vi "1A_AnalyzePulseTrain.vi"(0 "Waveform In":waveform(dbl)={"t0"=timestamp(3433165898.5470004 s since 1904-01-01), "dt"=1e-05, "Y"=array[4250 elements]}, 5 "Repetitions in the Input Waveform":i32, 7 "Pulse Characteristics":T2={"Pulses per Cycle"=2, "Load Resistance (Ohms)"=750.0, "Krec Value"=2, "Recovery Mode (T=Active)"=TRUE, "Target Stim Currents (Amps)"=[]}) -> (2 "Avg. CBC Width":dbl format="%0.6f", 3 "Avg. CBC Amplitude":dbl format="%0.2f", 4 "Stim PW":dbl[](array[numeric]), 6 "Stim Amplitude":dbl[](array[numeric]), 8 "Interphase Delay":dbl[](array[numeric]) format="%#.6g", 10 "Recovery PW":dbl[](array[numeric]), 12 "Waveform Parameters":T1, 13 "Frequency":dbl, 14 "Recovery Holdoff":dbl[](array[numeric]), 15 "Recovery Amplitude":dbl[](array[numeric]))   [LabVIEW 2010]
uses:
  Pulse Train Parameters.ctl
  <vilib>/measure/mamon.llb/Trigger Detection for 1 Channel.vi
  <vilib>/measure/NI_MAPro.lvlib
  <vilib>/Analysis/NI_AALBase.lvlib
panel:
  out "Normalized Waveform":waveform(dbl)(graph)
  # "The input waveform should be a capture of the STIM chip output\n(before the cap) when the output is held at 1/2 HVDD by the\nLoad Resistance.  This ensures that passive recovery and CBC\npulses are captured, because they look like pulses pulled to GND."
  # "The elements in these arrays correspond to the pulses per cycle.\nThey are the averages over all the repetitions in the waveform."
  # "Enter Target Current\nfor each in array below"
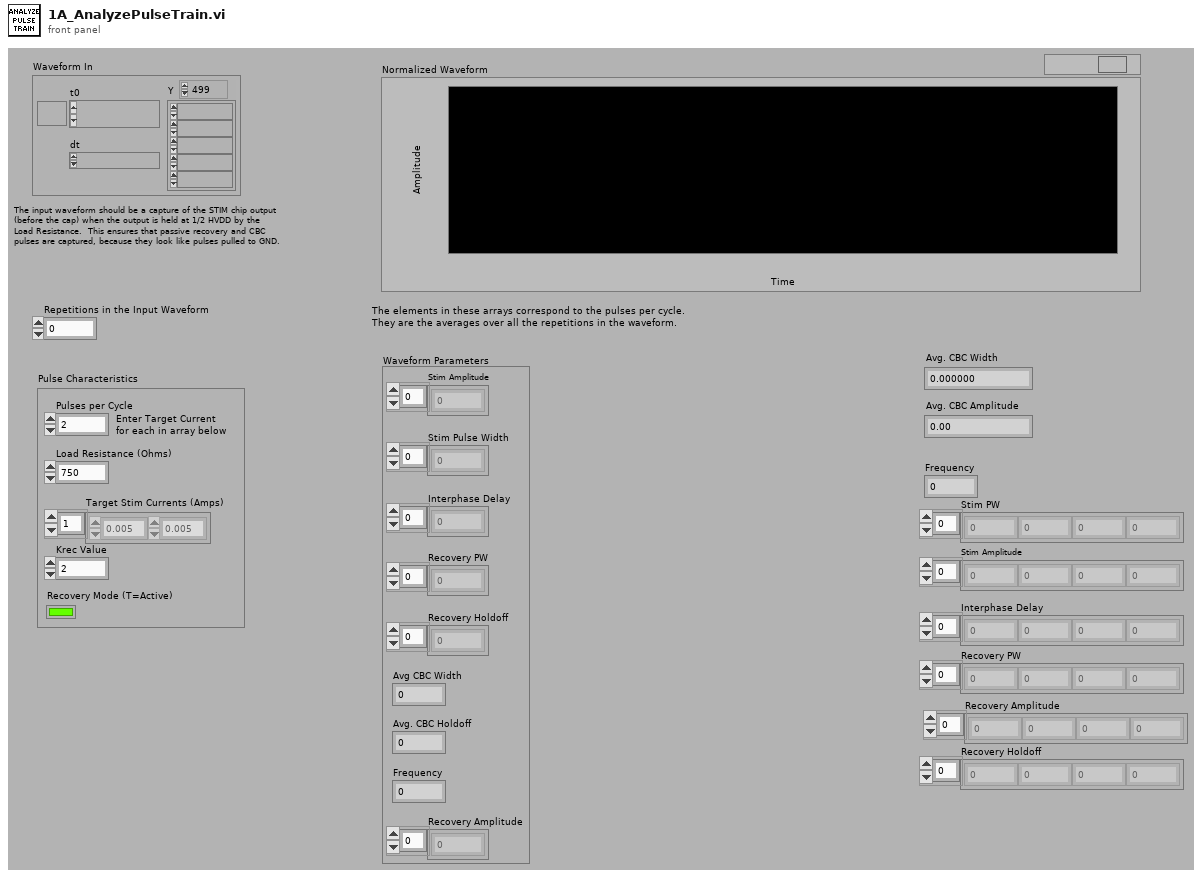
[diagram p1: front panel]
types:
  T1 = typedef "Pulse Train Parameters.ctl" = cluster{"Stim Amplitude":dbl[], "Stim Pulse Width":dbl[], "Interphase Delay":dbl[], "Recovery PW":dbl[], "Recovery Holdoff":dbl[], "Avg CBC Width":dbl, "Frequency":dbl, "Avg. CBC Holdoff":dbl, "Recovery Amplitude":dbl[]}
  T2 = cluster{"Pulses per Cycle":i32, "Load Resistance (Ohms)":dbl, "Krec Value":i32, "Recovery Mode (T=Active)":bool, "Target Stim Currents (Amps)":dbl[]}
  T3 = cluster{"trigger slope":u16, "Trigger Level":dbl}[]
  T4 = cluster{"trigger slope":u16, "Trigger Level":dbl}
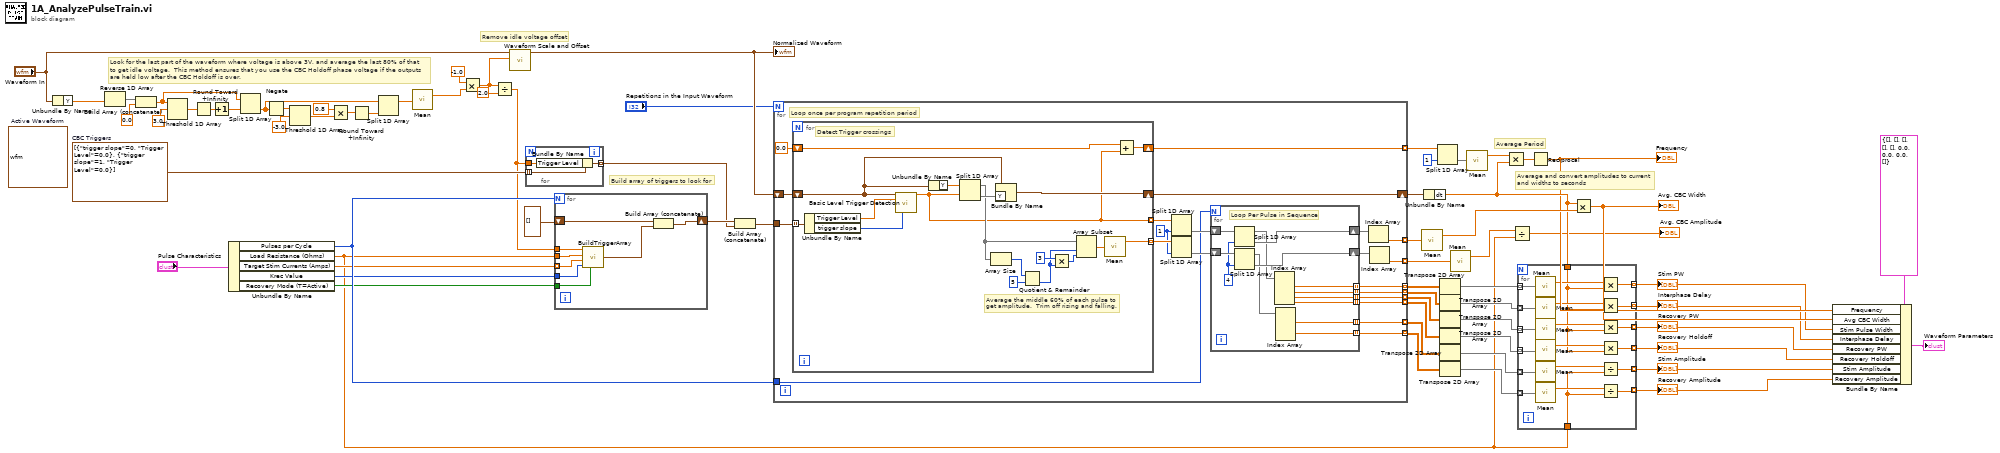
[diagram p0: block diagram]
diagram:
  (unwired) waveform(dbl) {"t0"=timestamp(3418839276.250478 s since 1904-01-01), "dt"=1e-06, "Y"=[5.0, 5.0, 9.0, 9.0, 9.0, 9.0, 9.0, 9.0, 9.0, 9.0, 5.0, 5.0, 5.0, 3.0, 3.0, 3.0, 3.0, 3.0, 3.0, 3.0, 3.0, 3.0, 3.0, 3.0, 3.0, 3.0, 3.0, 3.0, 3.0, 5.0, 5.0, 5.0, 5.0, 8.0, 8.0, 8.0, 8.0, 8.0, 8.0, 8.0, 8.0, 5.0, 5.0, 5.0, 3.0, 3.0, 3.0, 3.0, 3.0, 3.0, 3.0, 3.0, 3.0, 3.0, 3.0, 3.0, 3.0, 3.0, 3.0, 3.0, 5.0, 5.0, 5.0, 5.0, 0.0, 0.0, 0.0, 0.0, 0.0, 5.0, 5.0, 5.0, 5.0, 5.0, 5.0, 5.0, 5.0, 5.0, 5.0, 5.0, 5.0, 5.0, 5.0, 5.0, 5.0, 5.0, 5.0, 5.0, 5.0, 5.0, 5.0, 5.0, 5.0, 5.0, 5.0, 5.0, 5.0, 5.0, 5.0, 5.0, 5.0, 5.0, 9.0, 9.0, 9.0, 9.0, 9.0, 9.0, 9.0, 9.0, 5.0, 5.0, 5.0, 3.0, 3.0, 3.0, 3.0, 3.0, 3.0, 3.0, 3.0, 3.0, 3.0, 3.0, 3.0, 3.0, 3.0, 3.0, 3.0, 5.0, 5.0, 5.0, 5.0, 8.0, 8.0, 8.0, 8.0, 8.0, 8.0, 8.0, 8.0, 5.0, 5.0, 5.0, 3.0, 3.0, 3.0, 3.0, 3.0, 3.0, 3.0, 3.0, 3.0, 3.0, 3.0, 3.0, 3.0, 3.0, 3.0, 3.0, 5.0, 5.0, 5.0, 5.0, 0.0, 0.0, 0.0, 0.0, 0.0, 5.0, 5.0, 5.0, 5.0, 5.0, 5.0, 5.0, 5.0, 5.0, 5.0, 5.0, 5.0, 5.0, 5.0, 5.0, 5.0, 5.0, 5.0, 5.0, 5.0, 5.0, 5.0, 5.0, 5.0, 5.0, 5.0, 5.0, 5.0, 5.0, 5.0, 5.0, 5.0, 5.0, 9.0, 9.0, 9.0, 9.0, 9.0, 9.0, 9.0, 9.0, 5.0, 5.0, 5.0, 3.0, 3.0, 3.0, 3.0, 3.0, 3.0, 3.0, 3.0, 3.0, 3.0, 3.0, 3.0, 3.0, 3.0, 3.0, 3.0, 5.0, 5.0, 5.0, 5.0, 8.0, 8.0, 8.0, 8.0, 8.0, 8.0, 8.0, 8.0, 5.0, 5.0, 5.0, 3.0, 3.0, 3.0, 3.0, 3.0, 3.0, 3.0, 3.0, 3.0, 3.0, 3.0, 3.0, 3.0, 3.0, 3.0, 3.0, 5.0, 5.0, 5.0, 5.0, 0.0, 0.0, 0.0, 0.0, 0.0, 5.0, 5.0, 5.0, 5.0, 5.0, 5.0, 5.0, 5.0, 5.0, 5.0, 5.0, 5.0, 5.0, 5.0, 5.0, 5.0, 5.0, 5.0, 5.0, 5.0, 5.0, 5.0, 5.0, 5.0, 5.0, 5.0, 5.0, 5.0, 5.0, 5.0, 5.0, 5.0, 5.0, 9.0, 9.0, 9.0, 9.0, 9.0, 9.0, 9.0, 9.0, 5.0, 5.0, 5.0, 3.0, 3.0, 3.0, 3.0, 3.0, 3.0, 3.0, 3.0, 3.0, 3.0, 3.0, 3.0, 3.0, 3.0, 3.0, 3.0, 5.0, 5.0, 5.0, 5.0, 8.0, 8.0, 8.0, 8.0, 8.0, 8.0, 8.0, 8.0, 5.0, 5.0, 5.0, 3.0, 3.0, 3.0, 3.0, 3.0, 3.0, 3.0, 3.0, 3.0, 3.0, 3.0, 3.0, 3.0, 3.0, 3.0, 3.0, 5.0, 5.0, 5.0, 5.0, 0.0, 0.0, 0.0, 0.0, 0.0, 5.0, 5.0, 5.0, 5.0, 5.0, 5.0, 5.0, 5.0, 5.0, 5.0, 5.0, 5.0, 5.0, 5.0, 5.0, 5.0, 5.0, 5.0, 5.0, 5.0, 5.0, 5.0, 5.0, 5.0, 5.0, 5.0, 5.0, 5.0, 5.0, 5.0, 5.0, 5.0, 5.0, 9.0, 9.0, 9.0, 9.0, 9.0, 9.0, 9.0, 9.0, 5.0, 5.0, 5.0, 3.0, 3.0, 3.0, 3.0, 3.0, 3.0, 3.0, 3.0, 3.0, 3.0, 3.0, 3.0, 3.0, 3.0, 3.0, 3.0, 5.0, 5.0, 5.0, 5.0, 8.0, 8.0, 8.0, 8.0, 8.0, 8.0, 8.0, 8.0, 5.0, 5.0, 5.0, 3.0, 3.0, 3.0, 3.0, 3.0, 3.0, 3.0, 3.0, 3.0, 3.0, 3.0, 3.0, 3.0, 3.0, 3.0, 3.0, 5.0, 5.0, 5.0, 5.0, 0.0, 0.0, 0.0, 0.0, 0.0, 5.0, 5.0, 5.0, 5.0, 5.0, 5.0, 5.0, 5.0, 5.0, 5.0, 5.0, 5.0, 5.0, 5.0, 5.0, 5.0, 5.0, 5.0, 5.0, 5.0, 5.0, 5.0, 5.0, 5.0, 5.0, 5.0, 5.0, 5.0, 5.0, 5.0, 5.0, 5.0, 5.0, 5.0]}  # Active Waveform
  w64 = T3 [{"trigger slope"=0, "Trigger Level"=0.0}, {"trigger slope"=1, "Trigger Level"=0.0}]  # CBC Triggers
  # "Look for the last part of the waveform where voltage is above 3V, and average the last 80% of that\nto get idle voltage.  This method ensures that you use the CBC Holdoff phase voltage if the outputs\nare held low after the CBC Holdoff is over."
  # "Average Period"
  # "Average and convert amplitudes to current\nand widths to seconds"
  # "Build array of triggers to look for"
  # "Remove idle voltage offset"
  n1 = Unbundle By Name("Waveform In") -> ("Y"=w2:dbl[])
  n2 = Reverse 1D Array(array=w2) -> (reversed array=w17:dbl[])
  n3 = Build Array (concatenate)(w17, 0.0 ("y")) -> (w12:dbl[])
  n4 = Threshold 1D Array(2:3.0 ("y"), 3:w12) -> (0:w14:dbl)  [unwired: 1 in]
  n5 = Round Toward +Infinity(x=w14) -> (ceil(x): smallest int >= x=w13:dbl)
  n6 = Increment(x=w13) -> (x+1=w3:dbl)
  n7 = Unbundle By Name("Pulse Characteristics") -> ("Pulses per Cycle"=w44:i32, "Load Resistance (Ohms)"=w35:dbl, "Target Stim Currents (Amps)"=w41:dbl[], "Krec Value"=w40:i32, "Recovery Mode (T=Active)"=w42:bool)
  n8 = Split 1D Array(array=w12, index=w3) -> (second subarray=w5:dbl[])  [unwired: 1 out]
  n9 = Negate(x=w5) -> (-x=w10:dbl[])
  n10 = Threshold 1D Array(2:-3.0 ("y"), 3:w10) -> (0:w9:dbl)  [unwired: 1 in]
  n11 = Multiply(x=0.8, y=w9) -> (x*y=w7:dbl)
  n12 = Round Toward +Infinity(x=w7) -> (ceil(x): smallest int >= x=w6:dbl)
  n13 = Split 1D Array(array=w5, index=w6) -> (first subarray=w4:dbl[])  [unwired: 1 out]
  n14 = call <vilib>:"Mean.vi"("X"=w4) -> ("mean"=w1:dbl)  [unwired: 1 out]
  n15 = Multiply(x=-1.0, y=w1) -> (x*y=w63:dbl)
  n16 = Divide(x=w63, y=2.0) -> (x/y=w43:dbl)
  n17 = call <vilib>:"Waveform Scale and Offset.vi"("offset"=w63, "waveform in"="Waveform In") -> ("waveform out"=w59:waveform(dbl))  [unwired: 8 in, 1 out]
  "Normalized Waveform" <- w59
  n18 = for {
    tunnel: w64 -> [w72] mode=indexing
    tunnel: w43 -> [w71]
    tunnel: [w70] -> w61 mode=indexing
    n19 = Bundle By Name(cluster=w72, "Trigger Level"=w71) -> (w70:T4)
  }
  n20 = for {
    N: w44 -> [_]
    shift-right: [w80] -> w65
    shift-left: T3 [] -> [w79]
    tunnel: w43 -> [w78]
    tunnel: w42 -> [w77]
    tunnel: w35 -> [w76]
    tunnel: w41 -> [w75] mode=indexing
    tunnel: w40 -> [w74]
    n21 = call "BuildTriggerArray.vi"("CBC Trigger Level"=w78, "Load Resistance (Ohms)"=w76, "Target Stim Current (Amps)"=w75, "Krec Value"=w74, "Recovery Mode (T=Active)"=w77) -> ("Pulse Triggers"=w73:T3)
    n22 = Build Array (concatenate)(w79, w73) -> (w80:T3)
  }
  n23 = Build Array (concatenate)(w65, w61) -> (w60:T3)
  n24 = for {
    N: "Repetitions in the Input Waveform" -> [_]
    tunnel: w60 -> [w101]
    shift-right: [w97] -> w38
    shift-left: w59 -> [w100]
    tunnel: w44 -> [w94]
    tunnel: [w91] -> w58 mode=indexing
    tunnel: [w90] -> w57 mode=indexing
    tunnel: [w89] -> w56 mode=indexing
    tunnel: [w88] -> w55 mode=indexing
    tunnel: [w87] -> w54 mode=indexing
    tunnel: [w86] -> w53 mode=indexing
    tunnel: [w85] -> w52 mode=indexing
    tunnel: [w84] -> w51 mode=indexing
    tunnel: [w81] -> w34 mode=indexing
    w98 = 1 ("index")
    # "Loop once per program repetition period"
    n25 = for {
      tunnel: w101 -> [w132] mode=indexing
      shift-right: [w118] -> w97
      shift-left: w100 -> [w127]
      tunnel: [w119] -> w99 mode=indexing
      tunnel: [w115] -> w82 mode=indexing
      shift-right: [w117] -> w81
      shift-left: 0.0 -> [w116]
      # "Detect Trigger crossings"
      # "Average the middle 60% of each pulse to\nget amplitude.  Trim off rising and falling."
      n26 = Unbundle By Name(w132) -> ("Trigger Level"=w131:dbl, "trigger slope"=w130:u16)
      n27 = call-poly <vilib>:"Basic Level Trigger Detection.vi"("signal in"=w127, "level"=w131, "trigger slope"=w130) -> ("trigger location"=w115:dbl)  [unwired: 10 in, 2 out]
      n28 = Unbundle By Name(w127) -> ("Y"=w129:dbl[])
      n29 = Split 1D Array(array=w129, index=w115) -> (first subarray=w121:dbl[], second subarray=w128:dbl[])
      n30 = Array Size(array=w121) -> (size(s)=w126:i32)
      n31 = Bundle By Name(cluster=w127, "Y"=w128) -> (w118:waveform(dbl))
      n32 = Quotient & Remainder(x=w126, y=5) -> (floor(x/y)=w123:i32)  [unwired: 1 out]
      n33 = Multiply(x=3, y=w123) -> (x*y=w122:i32)
      n34 = Array Subset(array=w121, index=w123, length=w122) -> (w120:dbl[])
      n35 = call <vilib>:"Mean.vi"("X"=w120) -> ("mean"=w119:dbl)  [unwired: 1 out]
      n36 = Add(x=w116, y=w115) -> (x+y=w117:dbl)
    }
    n37 = Split 1D Array(array=w82, index=w98) -> (second subarray=w96:dbl[])  [unwired: 1 out]
    n38 = Split 1D Array(array=w99, index=w98) -> (second subarray=w95:dbl[])  [unwired: 1 out]
    n39 = for {
      N: w94 -> [_]
      shift-right: [w112] -> w93
      shift-left: w96 -> [w114]
      shift-right: [w111] -> w92
      shift-left: w95 -> [w113]
      tunnel: [w108] -> w89 mode=indexing
      tunnel: [w107] -> w88 mode=indexing
      tunnel: [w106] -> w87 mode=indexing
      tunnel: [w105] -> w86 mode=indexing
      tunnel: [w104] -> w85 mode=indexing
      tunnel: [w103] -> w84 mode=indexing
      w102 = 4 ("index")
      # "Loop Per Pulse in Sequence"
      n40 = Split 1D Array(array=w114, index=w102) -> (first subarray=w110:dbl[], second subarray=w112:dbl[])
      n41 = Split 1D Array(array=w113, index=w102) -> (first subarray=w109:dbl[], second subarray=w111:dbl[])
      n42 = Index Array(array=w110) -> (element #1=w108:dbl, element #2=w107:dbl, element #3=w106:dbl, element #4=w105:dbl)  [unwired: 4 in]
      n43 = Index Array(array=w109) -> (element #1=w104:dbl, element #3=w103:dbl)  [unwired: 4 in, 2 out]
    }
    n44 = Index Array(array=w93) -> (element=w91:dbl)  [unwired: 1 in]
    n45 = Index Array(array=w92) -> (element=w90:dbl)  [unwired: 1 in]
  }
  n46 = call <vilib>:"Mean.vi"("X"=w58) -> ("mean"=w37:dbl)  [unwired: 1 out]
  n47 = Unbundle By Name(w38) -> ("dt"=w31:dbl)
  n48 = Split 1D Array(array=w34, index=1) -> (second subarray=w33:dbl[])  [unwired: 1 out]
  n49 = Transpose 2D Array(2D array=w56) -> (transposed array=w50:dbl[][])
  n50 = Transpose 2D Array(2D array=w55) -> (transposed array=w49:dbl[][])
  n51 = Transpose 2D Array(2D array=w54) -> (transposed array=w48:dbl[][])
  n52 = Transpose 2D Array(2D array=w53) -> (transposed array=w47:dbl[][])
  n53 = Transpose 2D Array(2D array=w52) -> (transposed array=w46:dbl[][])
  n54 = Transpose 2D Array(2D array=w51) -> (transposed array=w45:dbl[][])
  n55 = call <vilib>:"Mean.vi"("X"=w57) -> ("mean"=w36:dbl)  [unwired: 1 out]
  n56 = call <vilib>:"Mean.vi"("X"=w33) -> ("mean"=w32:dbl)  [unwired: 1 out]
  n57 = Multiply(x=w32, y=w31) -> (x*y=w30:dbl)
  n58 = Divide(x=w36, y=w35) -> (x/y=→"Avg. CBC Amplitude":dbl)
  n59 = for {
    tunnel: w50 -> [w152] mode=indexing
    tunnel: w49 -> [w151] mode=indexing
    tunnel: w48 -> [w150] mode=indexing
    tunnel: w47 -> [w149] mode=indexing
    tunnel: w46 -> [w148] mode=indexing
    tunnel: w45 -> [w147] mode=indexing
    tunnel: [w146] -> w24 mode=indexing
    tunnel: [w145] -> w23 mode=indexing
    tunnel: [w144] -> w22 mode=indexing
    tunnel: [w143] -> w21 mode=indexing
    tunnel: [w142] -> w20 mode=indexing
    tunnel: [w141] -> w19 mode=indexing
    tunnel: w31 -> [w134]
    tunnel: w35 -> [w133]
    n60 = call <vilib>:"Mean.vi"("X"=w152) -> ("mean"=w139:dbl)  [unwired: 1 out]
    n61 = call <vilib>:"Mean.vi"("X"=w151) -> ("mean"=w138:dbl)  [unwired: 1 out]
    n62 = call <vilib>:"Mean.vi"("X"=w150) -> ("mean"=w137:dbl)  [unwired: 1 out]
    n63 = call <vilib>:"Mean.vi"("X"=w149) -> ("mean"=w136:dbl)  [unwired: 1 out]
    n64 = call <vilib>:"Mean.vi"("X"=w148) -> ("mean"=w135:dbl)  [unwired: 1 out]
    n65 = call <vilib>:"Mean.vi"("X"=w147) -> ("mean"=w140:dbl)  [unwired: 1 out]
    n66 = Multiply(x=w139, y=w134) -> (x*y=w146:dbl)
    n67 = Multiply(x=w138, y=w134) -> (x*y=w145:dbl)
    n68 = Multiply(x=w137, y=w134) -> (x*y=w144:dbl)
    n69 = Multiply(x=w136, y=w134) -> (x*y=w143:dbl)
    n70 = Divide(x=w135, y=w133) -> (x/y=w142:dbl)
    n71 = Divide(x=w140, y=w133) -> (x/y=w141:dbl)
  }
  "Stim PW" <- w24
  "Interphase Delay" <- w23
  "Recovery PW" <- w22
  "Recovery Holdoff" <- w21
  "Stim Amplitude" <- w20
  "Recovery Amplitude" <- w19
  n72 = Reciprocal(x=w30) -> (1/x=w27:dbl)
  "Frequency" <- w27
  n73 = Multiply(x=w31, y=w37) -> (x*y=w26:dbl)
  "Avg. CBC Width" <- w26
  n74 = Bundle By Name(cluster=T1 {"Stim Amplitude"=[], "Stim Pulse Width"=[], "Interphase Delay"=[], "Recovery PW"=[], "Recovery Holdoff"=[], "Avg CBC Width"=0.0, "Frequency"=0.0, "Avg. CBC Holdoff"=0.0, "Recovery Amplitude"=[]} ("Pulse Train Parameters"), "Frequency"=w27, "Avg CBC Width"=w26, "Stim Pulse Width"=w24, "Interphase Delay"=w23, "Recovery PW"=w22, "Recovery Holdoff"=w21, "Stim Amplitude"=w20, "Recovery Amplitude"=w19) -> (→"Waveform Parameters":T1)
